vi "Update Info.vi"(8 "error in (no error)":errorcluster, 9 "Get All Info":bool, 11 "CIF_UI in":refnum<class "CIF_Manager_UI.lvclass">) -> (0 "error out":errorcluster, 1 "Info":string)   [LabVIEW 2021, in "CIF_Manager_UI.lvclass"]
uses:
  CIF_Manager_UI.lvclass
  C:/Program Files/National Instruments/LabVIEW 2021/vi.lib/CIF Foundation/CIF Core/CIFUI/CIF_UI.lvclass
  <vilib>/CIF Foundation/CIF Core/CIFUI/CIF_UI.lvclass/CIF_UI.ctl
  <vilib>/CIF Foundation/CIF Core/CIFUI/Accessors/Read Manager gRPC ID.vi
  <vilib>/CIF Foundation/CIF Core/CIFUI/Accessors/Read Manager Connection.vi
  CIF_Manager_UI.lvclass/CIF_Manager_UI.ctl
  <vilib>/CIF Foundation/CIF Core/CIFPluginManager/gRPC/CIF_Manager_Client_Wrapper/CIFManagerClientWrapper.lvlib
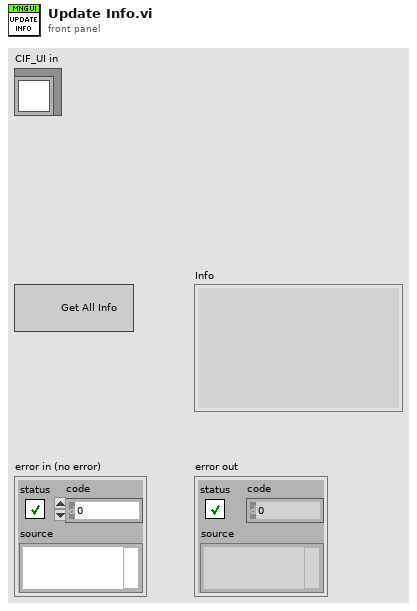
[diagram p1: front panel]
types:
  T1 = typedef "grpc-lvsupport-release.lvlib/grpcId.ctl" = u64
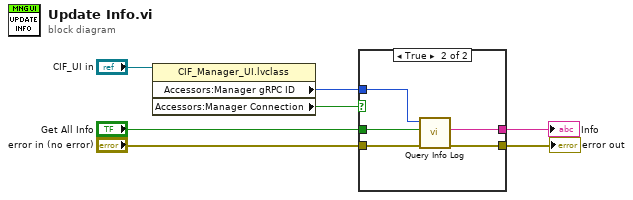
[diagram p0: block diagram]
diagram:
  n1 = property class="CIF_Manager_UI.lvclass"(reference="CIF_UI in") -> ("Accessors:Manager gRPC ID"=w1:T1, "Accessors:Manager Connection"=w2:bool)  [unwired: 1 in, 2 out]
  n2 = case shown="True" w2 {
    tunnel: "Get All Info" -> [_ w13]
    tunnel: [w8 w9] -> w6
    tunnel: [_ w12] -> w5
    tunnel: w1 -> [_ w11]
    tunnel: "error in (no error)" -> [w8 w10]
    frame False {
    }
    frame True {
      n3 = call <vilib>:"Query Info Log.vi"("error in"=w10, "query_all"=w13, "gRPC ID in"=w11) -> ("error out"=w9:errorcluster, "Info"=w12:string)  [unwired: 6 in, 1 out]
    }
  }
  "error out" <- w6
  "Info" <- w5
